vi "Read datatype.vi"(8 "error in (no error)":errorcluster, 11 "JSON Null in":refnum<class "JSON Null.lvclass">) -> (0 "error out":errorcluster, 2 "datatype":T1, 3 "JSON Null out":refnum<class "JSON Null.lvclass">)   [LabVIEW 2015, in "LVJSON.lvlib" / "JSON Null.lvclass"]
uses:
  JSON Null.lvclass
  JSON Types.ctl
  LVJSON.lvlib
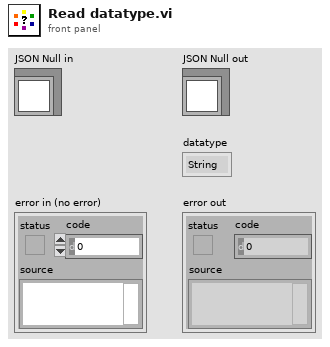
[diagram p1: front panel]
types:
  T1 = typedef "LVJSON.lvlib/JSON Types.ctl" = enum16{"String", "Numeric", "Boolean", "NULL", "Object", "1D Array", "Unknown"}
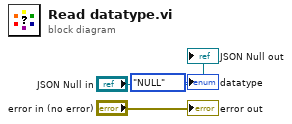
[diagram p0: block diagram]
diagram:
  "error out" <- "error in (no error)"
  "JSON Null out" <- "JSON Null in"
  "datatype" <- JSON_Types."NULL" ("datatype")
